vi "UI - Initiate Connection.vi"(8 "error in":errorcluster, 10 "Controller Address":string, 11 "Message Queue":refnum<queue>) -> (0 "error out":errorcluster, 1 "Connected?":bool)   [LabVIEW 2018]
uses:
  Message Queue/Message Cluster.ctl
  Message Queue/Message.ctl
  Controls/VTF Sensors.ctl
  Controls/Shared Variable References.ctl
  Globals/Global - Configuration Options.vi
  Globals/Global - UI Stream and Variable Connections.vi
  Message Queue/Message Queue.lvlib
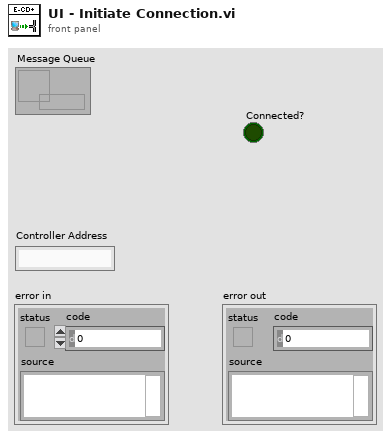
[diagram p1: front panel]
types:
  T1 = typedef "VTF Sensors.ctl" = cluster{"TJM Temp":dbl, "BrgM Temp":dbl, "Ambient Temp":dbl, "Vessel Temp":dbl}
  T2 = typedef "Message Queue.lvlib/Message Cluster.ctl" = cluster{"Message":T3, "Message Data":variant}
  T3 = typedef "Message Queue.lvlib/Message.ctl" = enum16{"Initialize", "Initialize UI Refs", "Disable Controls", "Enable UI Controls", "Connect RT", "Get Control Mode from RT", "Send Control Mode to UI", "Update Control Mode", "Get Config from RT", "Send Config to UI", "Update Parameters", "Change Parameters", "Calibrate Config", "Update Calibration", "Change Valve State", "Get Valve Status from RT", "Send Valve Status to UI", "Update Valve Status", "Inital UI Values", "Disconnect RT", "Close Connection", "Disconnect UI", "Run Mode", "Stop ALL", "Change Control Mode", "Skid Manual", "Computer Manual", "Step Automated", "Fully Automated", "Reset", "Critical Error", "Log-Only Error", "Non-Critical Error", "RT Error", "Update System Status", "Update DI Status", "Clear System Status", "Update Warning", "Clear Warning", "Upate Timeout", "Update Reset Status", "Waiting", "Verify Password", "Manual Cleaning Process", "Update Manual Cleaning Process", "Exit", "---Copy This Frame---"}
  T4 = typedef "Shared Variable References.ctl" = cluster{"CPU Usage":refnum<k21>, "Contiguous Memory":refnum<k21>, "VTF Sensors":refnum<k21>}
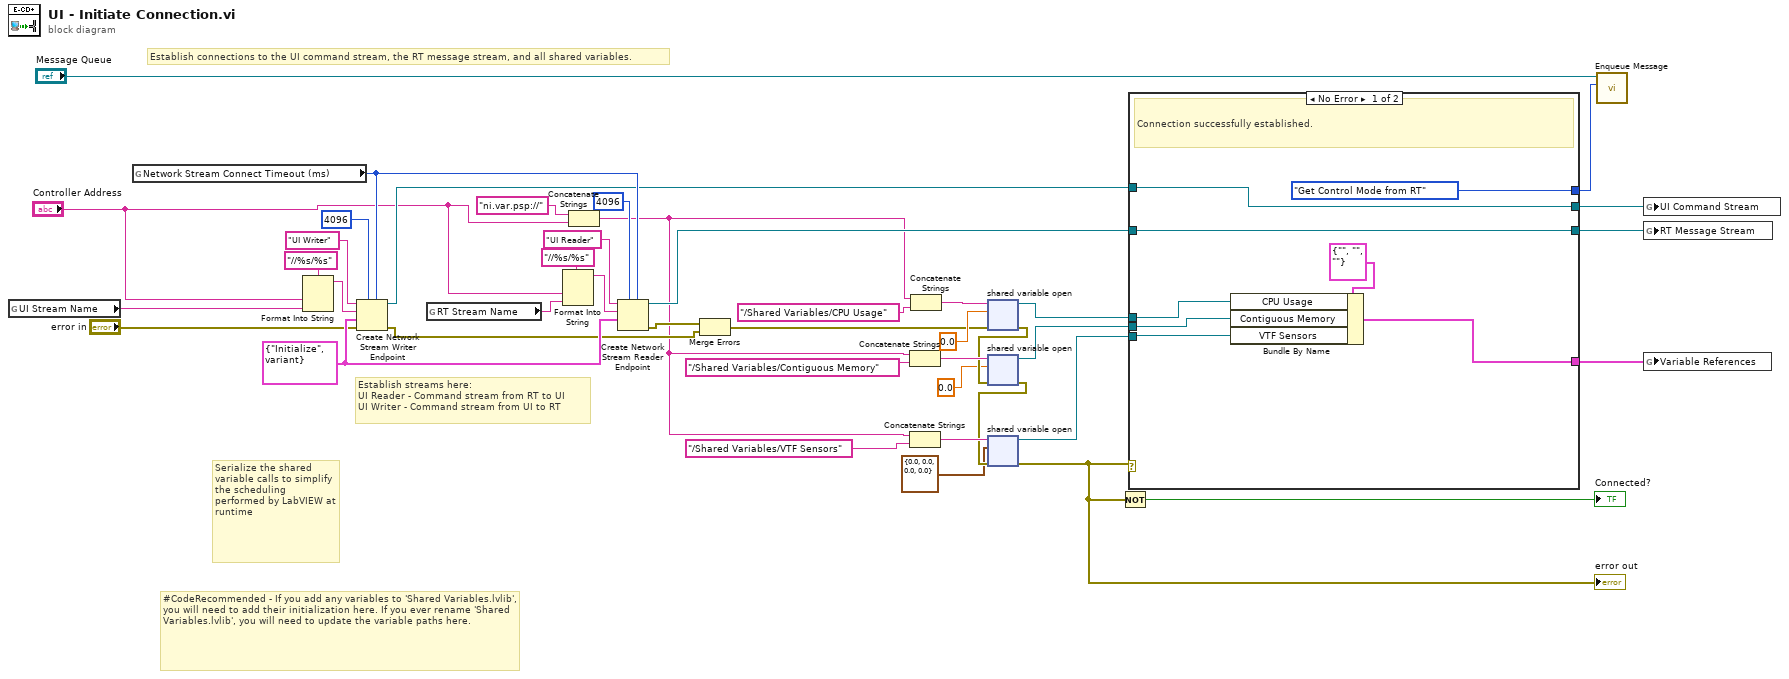
[diagram p0: block diagram]
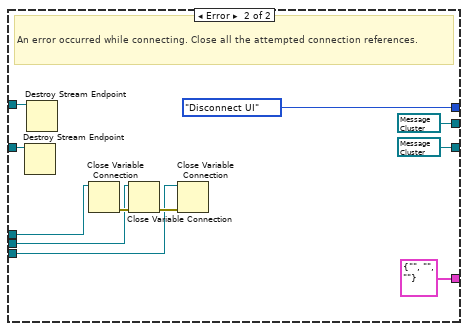
[diagram p2: hidden frame]
diagram:
  w33 = T2 {"Message"=enum."Initialize", "Message Data"=variant} ("Message Cluster")
  # "Establish connections to the UI command stream, the RT message stream, and all shared variables."
  # "#CodeRecommended - If you add any variables to 'Shared Variables.lvlib', you will need to add their initialization here. If you ever rename 'Shared Variables.lvlib', you will need to update the variable paths here."
  # "Establish streams here:\nUI Reader - Command stream from RT to UI\nUI Writer - Command stream from UI to RT"
  # "Serialize the shared variable calls to simplify the scheduling performed by LabVIEW at runtime"
  n1 = global read "Global - Configuration Options.vi" "UI Stream Name"() -> (w40:string)
  n2 = global read "Global - Configuration Options.vi" "Network Stream Connect Timeout (ms)"() -> (w32:i32)
  n3 = Format Into String(format string="//%s/%s", "Controller Address", w40) -> (resulting string=w39:string)  [unwired: 2 in, 1 out]
  n4 = Create Network Stream Writer Endpoint(5:w32, 7:4096 ("writer buffer size"), 8:"error in", 9:w33, 10:w39, 11:"UI Writer" ("writer name")) -> (0:w11:errorcluster, 3:w22:refnum<k21>)  [unwired: 1 in]
  n5 = global read "Global - Configuration Options.vi" "RT Stream Name"() -> (w37:string)
  n6 = Format Into String(format string="//%s/%s", "Controller Address", w37) -> (resulting string=w36:string)  [unwired: 2 in, 1 out]
  n7 = Concatenate Strings("ni.var.psp://", "Controller Address") -> (w5:string)
  n8 = Create Network Stream Reader Endpoint(5:w32, 7:4096 ("reader buffer size"), 9:w33, 10:w36, 11:"UI Reader" ("reader name")) -> (0:w12:errorcluster, 3:w21:refnum<k21>)  [unwired: 2 in]
  n9 = Merge Errors(w12, w11) -> (w13:errorcluster)
  n10 = Concatenate Strings(w5, "/Shared Variables/Contiguous Memory") -> (w26:string)
  n11 = Concatenate Strings(w5, "/Shared Variables/VTF Sensors") -> (w7:string)
  n12 = Concatenate Strings(w5, "/Shared Variables/CPU Usage") -> (w29:string)
  n13 = shared-variable-open(w29, w13, 0.0) -> (w24:refnum<k21>, w25:errorcluster)  [unwired: 1 in]
  n14 = shared-variable-open(w26, w25, 0.0) -> (w23:refnum<k21>, w4:errorcluster)  [unwired: 1 in]
  n15 = shared-variable-open(w7, w4, T1 {"TJM Temp"=0.0, "BrgM Temp"=0.0, "Ambient Temp"=0.0, "Vessel Temp"=0.0} ("VTF SENSORS")) -> (w1:refnum<k21>, w3:errorcluster)  [unwired: 1 in]
  "error out" <- w3
  n16 = Not(x=w3) -> (.not. x?=→"Connected?":bool)
  n17 = case shown="No Error" w3 {
    tunnel: w24 -> [w49 w58]
    tunnel: w23 -> [w48 w57]
    tunnel: w22 -> [w45 w60]
    tunnel: w21 -> [w46 w61]
    tunnel: [w47 T4 {"CPU Usage"="", "Contiguous Memory"="", "VTF Sensors"=""} ("Variable References")] -> w8
    tunnel: [w46 refnum<k21> refnum] -> w20
    tunnel: [w45 refnum<k21> refnum] -> w19
    tunnel: [Message."Get Control Mode from RT" ("Message") Message."Disconnect UI" ("Message")] -> w14
    tunnel: w1 -> [w43 w51]
    frame No Error {
      # "Connection successfully established."
      n18 = Bundle By Name(cluster=T4 {"CPU Usage"="", "Contiguous Memory"="", "VTF Sensors"=""} ("Variable References"), "CPU Usage"=w49, "Contiguous Memory"=w48, "VTF Sensors"=w43) -> (w47:T4)
    }
    frame Error {
      # "An error occurred while connecting. Close all the attempted connection references."
      n19 = Destroy Stream Endpoint(11:w61) -> ()  [unwired: 1 in, 1 out]
      n20 = Destroy Stream Endpoint(11:w60) -> ()  [unwired: 1 in, 1 out]
      n21 = Close Variable Connection(11:w58) -> (0:w59:errorcluster)  [unwired: 1 in]
      n22 = Close Variable Connection(8:w59, 11:w57) -> (0:w52:errorcluster)
      n23 = Close Variable Connection(8:w52, 11:w51) -> ()  [unwired: 1 out]
    }
  }
  n24 = call "Enqueue Message.vi"("Message"=w14, "Message Queue"="Message Queue") -> ()  [unwired: 8 in, 2 out]
  n25 = global write "Global - UI Stream and Variable Connections.vi" "UI Command Stream"(w19) -> ()
  n26 = global write "Global - UI Stream and Variable Connections.vi" "RT Message Stream"(w20) -> ()
  n27 = global write "Global - UI Stream and Variable Connections.vi" "Variable References"(w8) -> ()
